vi "Read.vi"(8 "error in (no error)":errorcluster, 11 "Boolean in":refnum<class "FPGA-Bus_SGL.lvclass">) -> (0 "error out":errorcluster, 2 "Numeric":T1, 3 "Boolean out":refnum<class "FPGA-Bus_SGL.lvclass">)   [LabVIEW 2021, in "FPGA-Bus_SGL.lvclass"]
uses:
  FPGA-Bus_SGL.lvclass
  Support/Value Type.ctl
  FPGA-Bus_SGL.lvclass/FPGA-Bus_SGL.ctl
  <vilib>/Utility/error.llb/Error Cluster From Error Code.vi
  <vilib>/rvi/errors/niLvFpgaAdjustHostInterfaceError.vi
  <vilib>/rvi/interface/nirviReadWriteControl/nirviReadWriteControl.xnode
  Support/FPGA Type.ctl
  NiFpgaLv.dll
  <vilib>/rvi/interface/Simulation/niFpgaSimulationCallBeginRW.vi
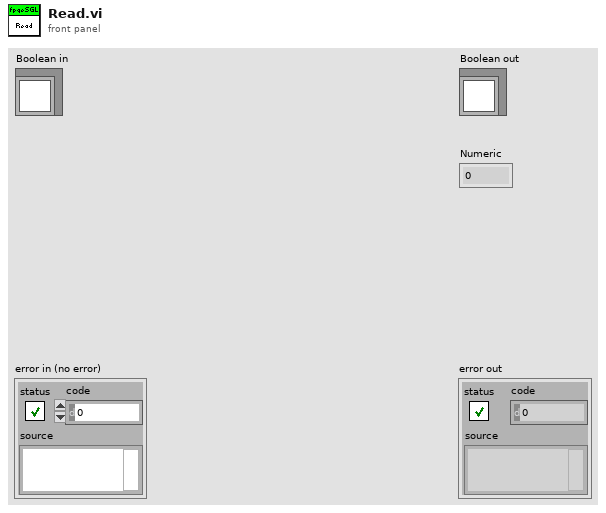
[diagram p1: front panel]
types:
  T1 = typedef "FPGA-Bus_SGL.lvclass/Value Type.ctl" = sgl
  T2 = typedef "FPGA-Bus_SGL.lvclass/FPGA Type.ctl" = refnum<k20>
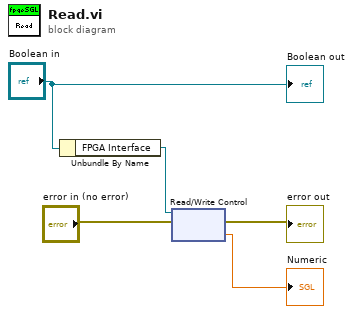
[diagram p0: block diagram]
diagram:
  n1 = Unbundle By Name("Boolean in") -> ("FPGA Interface"=w3:T2)
  n2 = xnode "Read/Write Control"("FPGA VI Reference In"=w3, "error in"="error in (no error)") -> ("error out"=→"error out":errorcluster, "Value"=→"Numeric":sgl)  [unwired: 1 out]
  "Boolean out" <- "Boolean in"
